vi "GetClassRef.vi"(0 "ClassReader in":refnum<class "ClassReader.lvclass">, 5 "error in (no error)":errorcluster) -> (14 "ClassReader out":refnum<class "ClassReader.lvclass">, 19 "error out":errorcluster)   [LabVIEW 2012, in "ClassReader.lvclass"]
uses:
  <resource>/Framework/Providers/Open_GDS/ClassProviders/Provider_BaseClassInterface/ClassReader_class/ClassReader.lvclass
  <resource>/Framework/Providers/Open_GDS/ClassProviders/Provider_BaseClassInterface/ClassReader_class/ClassReader.lvclass/ClassReader.ctl
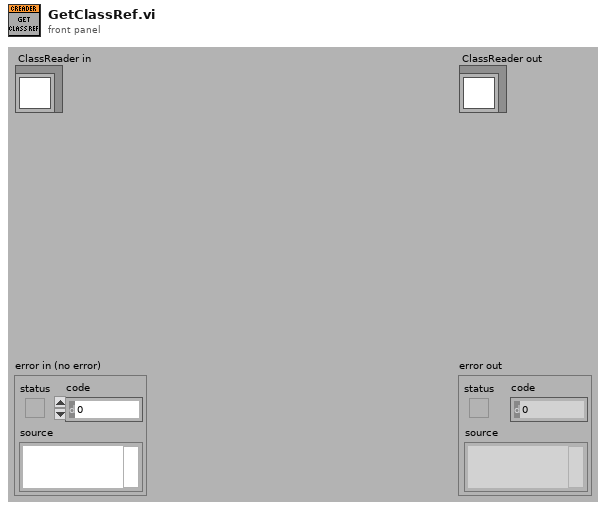
[diagram p1: front panel]
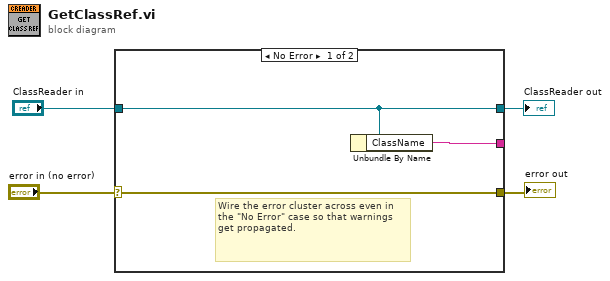
[diagram p0: block diagram]
diagram:
  n1 = case shown="No Error" "error in (no error)" {
    selector: "error in (no error)" -> [w7 w9]
    tunnel: [w7 w9] -> w3
    tunnel: [w6 w8] -> w1
    tunnel: "ClassReader in" -> [w6 w8]
    tunnel: [w5 _] -> _
    frame No Error {
      # "Wire the error cluster across even in the \"No Error\" case so that warnings get propagated."
      n2 = Unbundle By Name(w6) -> ("ClassName"=w5:string)
    }
    frame Error {
    }
  }
  "error out" <- w3
  "ClassReader out" <- w1
